vi "Write Pin.vi"(0 "Simulado in":refnum<class "Simulado.lvclass">, 5 "Port":dbl, 7 "Pin":dbl, 9 "Value":bool, 11 "error in (no error)":errorcluster) -> (4 "Simulado out":refnum<class "Simulado.lvclass">, 15 "error out":errorcluster)   [LabVIEW 2020, in "Simulado.lvclass"]
doc: "Escribe el valor del pin seleccionado"
uses:
  Simulado.lvclass
  Simulado.lvclass/Simulado.ctl
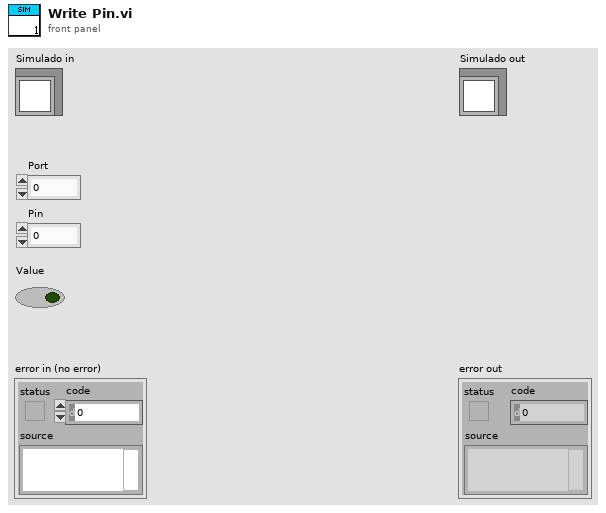
[diagram p1: front panel]
types:
  T1 = enum16{"Get Parameters", "Set Parameters", "Reset"}
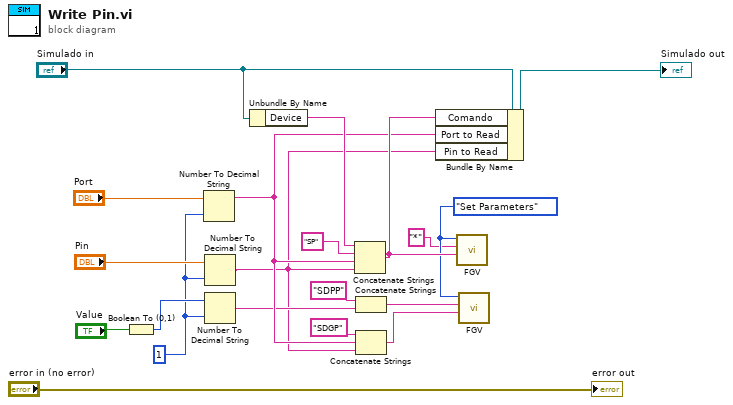
[diagram p0: block diagram]
diagram:
  w3 = i16 1 ("width (-)")
  w15 = T1."Set Parameters" ("Función")
  n1 = Boolean To (0,1)(Boolean="Value") -> (0, 1=w4:i16)
  n2 = Number To Decimal String(number="Port", width (-)=w3) -> (decimal integer string=w10:string)
  n3 = Number To Decimal String(number="Pin", width (-)=w3) -> (decimal integer string=w1:string)
  n4 = Number To Decimal String(number=w4, width (-)=w3) -> (decimal integer string=w2:string)
  n5 = Unbundle By Name("Simulado in") -> ("Device"=w18:string)
  n6 = Concatenate Strings(w18, "SP" ("string"), w10, w1) -> (w17:string)
  n7 = Concatenate Strings("SDPP" ("string"), w2) -> (w13:string)
  n8 = Concatenate Strings("SDGP" ("string"), w10, w1) -> (w11:string)
  n9 = Bundle By Name(cluster="Simulado in", "Comando"=w17, "Port to Read"=w10, "Pin to Read"=w1) -> (→"Simulado out":refnum<class "Simulado.lvclass">)
  n10 = call "FGV.vi"("Comandos"=w17, "Respuestas"="*", "Función"=w15) -> ()  [unwired: 8 in, 1 out]
  n11 = call "FGV.vi"("Comandos"=w11, "Respuestas"=w13, "Función"=w15) -> ()  [unwired: 8 in, 1 out]
  "error out" <- "error in (no error)"
